vi "oa_Segment XY Graph Sub.vi"(7 "Reset? (F)":bool, 8 "error in (no error)":errorcluster, 9 "Limit range":bool, 10 "Segment settings":T1={"X start"=0.0, "X interval"=50.0, "X end"=6000.0} {"X end" min=0.0 format="%.2f"; "X interval" format="%.2f"; "X start" min=0.0 format="%.2f"}, 11 "XY Graph":cluster{"time/rev/rpm":dbl[], "magnitude":dbl[]}) -> (0 "error out":errorcluster, 3 "XY Graph out":cluster{"time/rev/rpm":dbl[], "magnitude":dbl[]})   [LabVIEW 2017, in "SoundVib_Resampling.lvlib"]
uses:
  <vilib>/addons/Sound and Vibration/Order Analysis/Resample Order Tracking/SoundVib_Resampling.lvlib
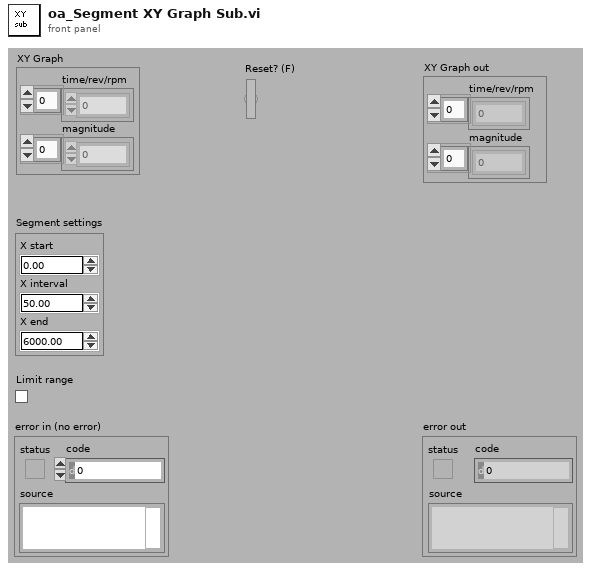
[diagram p1: front panel]
types:
  T1 = cluster{"X start":dbl, "X interval":dbl, "X end":dbl}
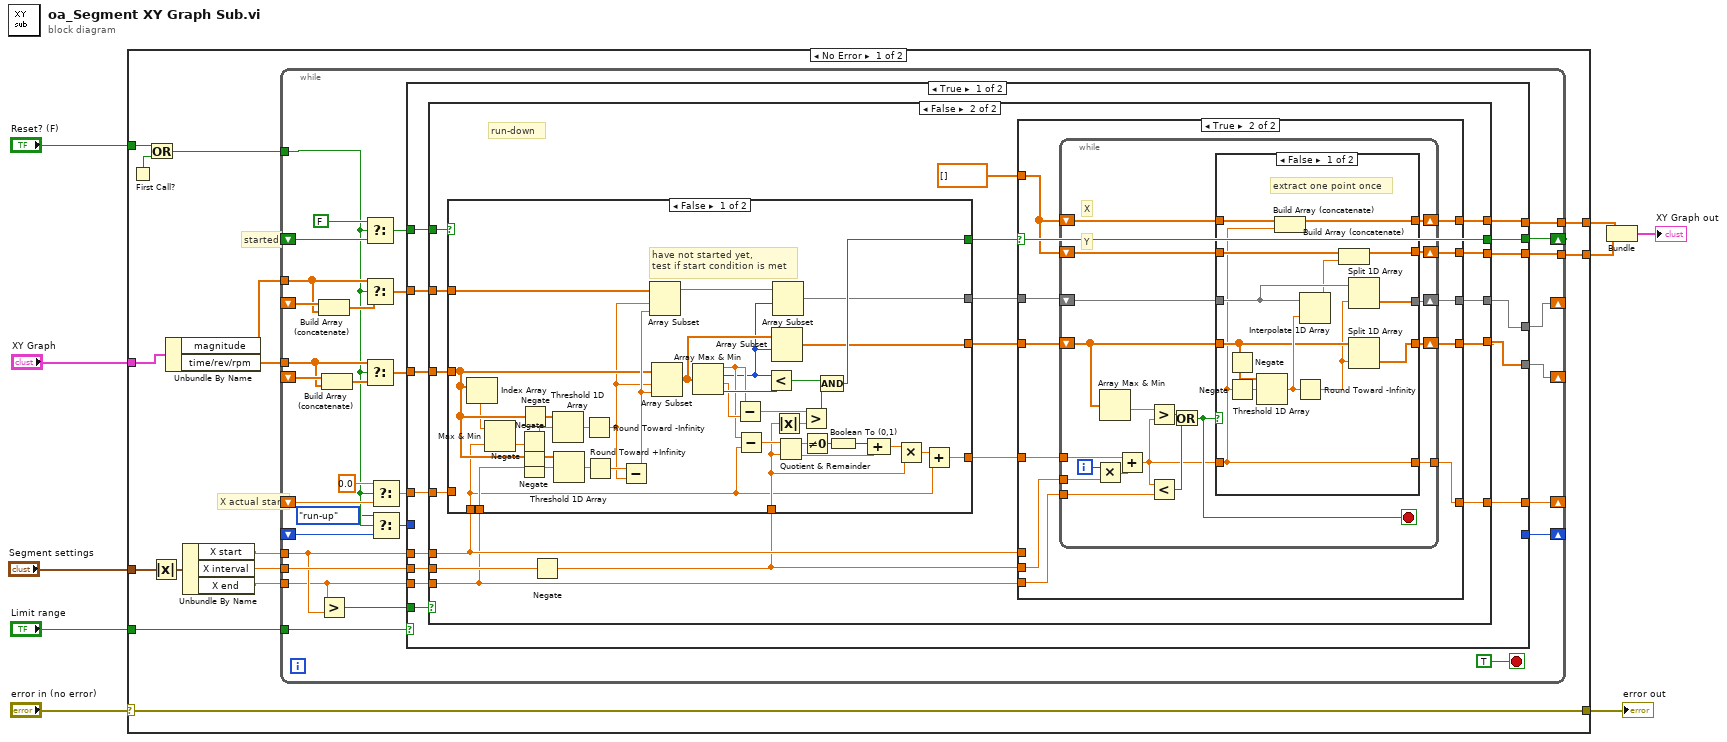
[diagram p0: block diagram]
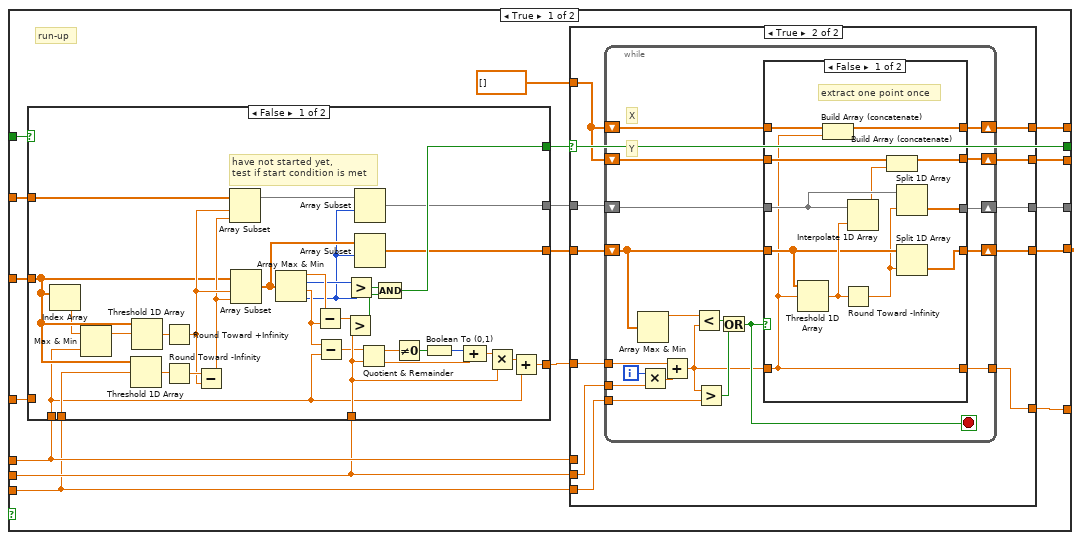
[diagram p2: hidden frame]
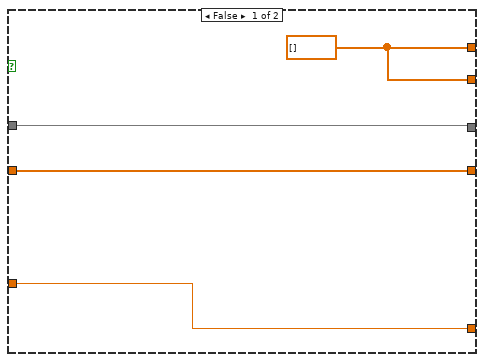
[diagram p3: hidden frame]
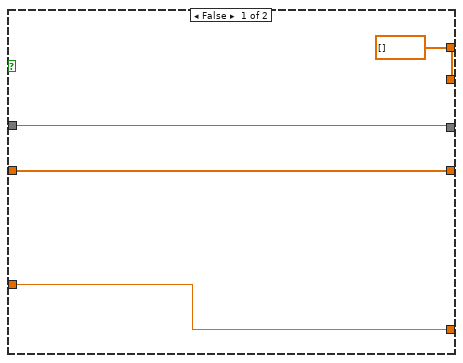
[diagram p6: hidden frame]
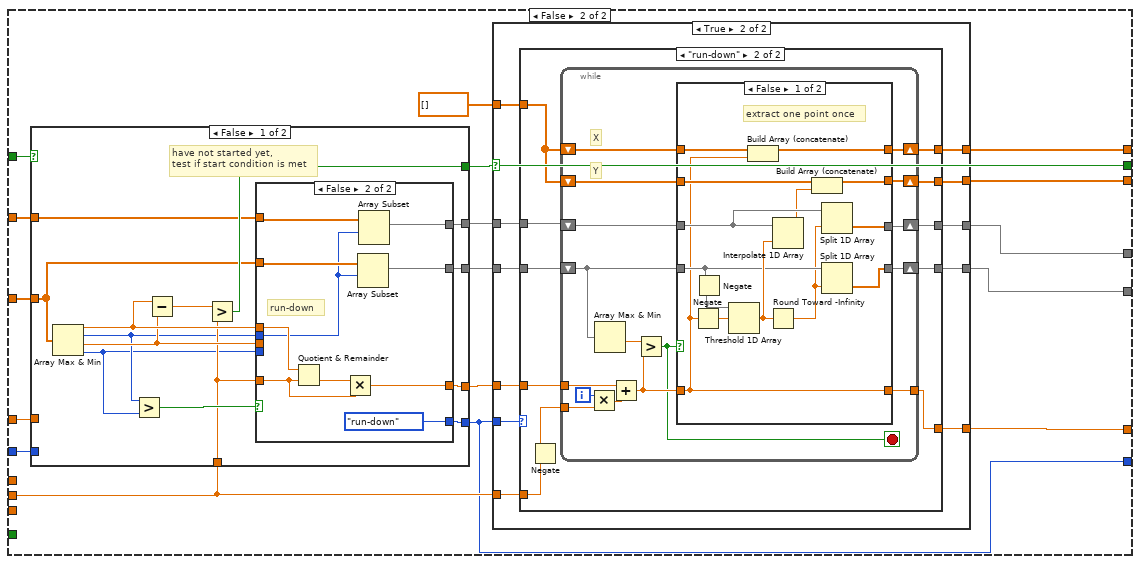
[diagram p9: hidden frame]
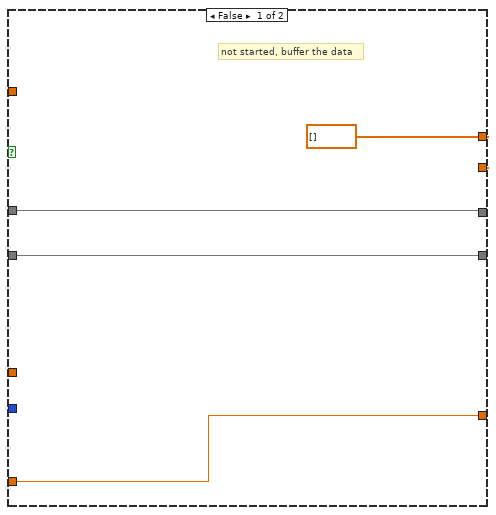
[diagram p10: hidden frame]
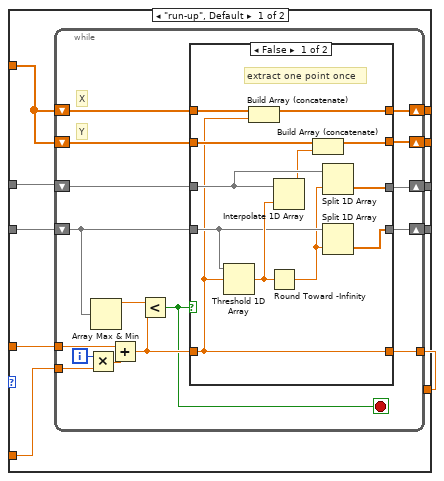
[diagram p11: hidden frame]
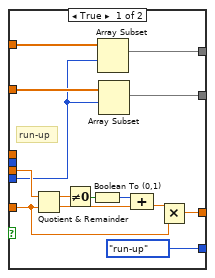
[diagram p14: hidden frame]
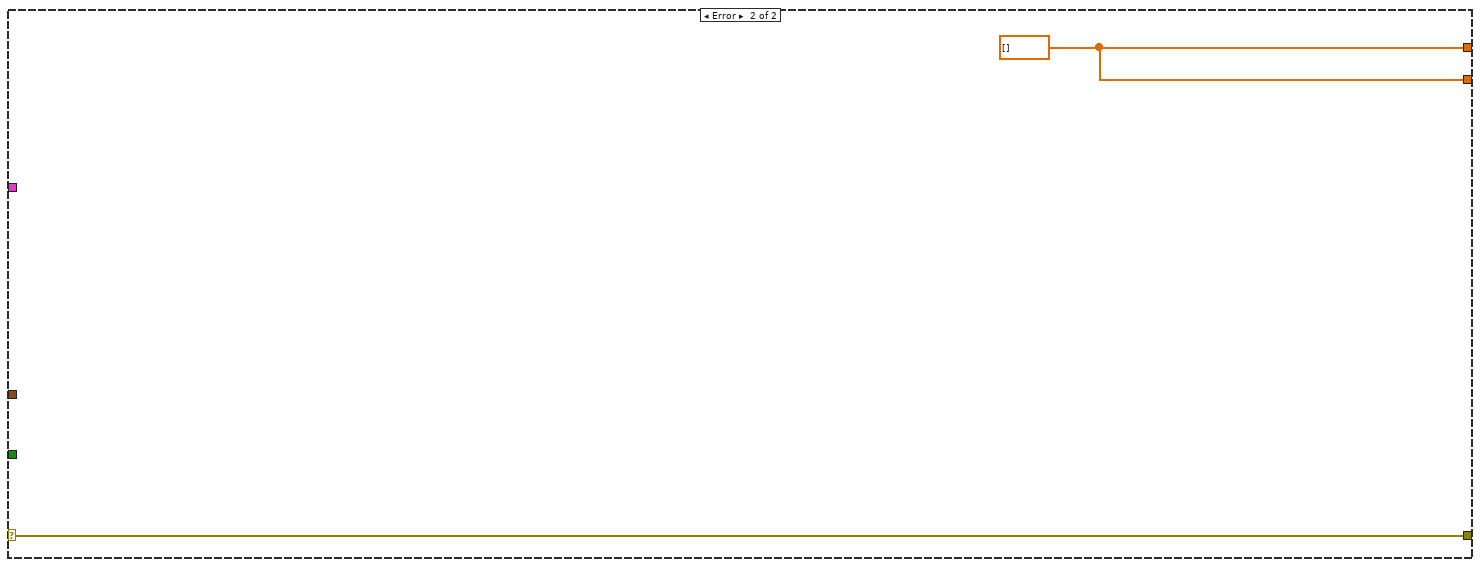
[diagram p16: hidden frame]
diagram:
  n1 = case shown="No Error" "error in (no error)" {
    selector: "error in (no error)" -> [w10 w451]
    tunnel: [w10 w451] -> w8
    tunnel: "Reset? (F)" -> [w24 _]
    tunnel: "Segment settings" -> [w17 _]
    tunnel: "Limit range" -> [w19 _]
    tunnel: "XY Graph" -> [w14 _]
    tunnel: [w12 w450] -> w3
    tunnel: [w11 w450] -> w2
    frame No Error {
      # "X actual start"
      # "started"
      n2 = First Call?() -> (First Call?: T/F=w23:bool)
      n3 = Or(x=w24, y=w23) -> (x .or. y?=w20:bool)
      n4 = Absolute Value(x=w17) -> (abs(x)=w16:T1)
      n5 = Unbundle By Name(w14) -> ("magnitude"=w13:dbl[], "time/rev/rpm"=w22:dbl[])
      n6 = Unbundle By Name(w16) -> ("X start"=w21:dbl, "X interval"=w18:dbl, "X end"=w15:dbl)
      n7 = while {
        tunnel: w22 -> [w52]
        tunnel: w21 -> [w37]
        shift-right: [w46] -> _
        shift-left: _ -> [w54]
        tunnel: w20 -> [w31]
        tunnel: w19 -> [w45]
        tunnel: w18 -> [w43]
        tunnel: w15 -> [w36]
        tunnel: w13 -> [w48]
        shift-right: [w47] -> _
        shift-left: _ -> [w50]
        shift-right: [w38] -> _
        shift-left: _ -> [w41]
        shift-right: [w33] -> _
        shift-left: _ -> [w34]
        shift-right: [w27] -> _
        shift-left: _ -> [w30]
        tunnel: [w26] -> w12
        tunnel: [w25] -> w11
        stop <- TRUE stop-if-true
        n8 = Build Array (concatenate)(w50, w48) -> (w49:dbl[])
        n9 = Greater?(x=w36, y=w37) -> (0:w44:bool)
        n10 = Build Array (concatenate)(w54, w52) -> (w53:dbl[])
        n11 = Select(t=FALSE, s=w31, f=w41) -> (s? t:f=w39:bool)
        n12 = Select(t=w48, s=w31, f=w49) -> (s? t:f=w42:dbl[])
        n13 = Select(t=w52, s=w31, f=w53) -> (s? t:f=w51:dbl[])
        n14 = Select(t=0.0, s=w31, f=w34) -> (s? t:f=w32:dbl)
        n15 = Select(t=enum16{"run-up", "run-down"}."run-up" ("process control"), s=w31, f=w30) -> (s? t:f=w28:enum16{"run-up", "run-down"})
        n16 = case shown="True" w45 {
          tunnel: w51 -> [w68 w300]
          tunnel: w42 -> [w62 w301]
          tunnel: [w57 w292] -> w47
          tunnel: [w56 w291] -> w46
          tunnel: w44 -> [w69 _]
          tunnel: w43 -> [w67 w294]
          tunnel: w39 -> [w66 w302]
          tunnel: [w65 w290] -> w38
          tunnel: w37 -> [w64 _]
          tunnel: w36 -> [w63 _]
          tunnel: w32 -> [w61 w299]
          tunnel: [w60 w289] -> w33
          tunnel: w28 -> [_ w298]
          tunnel: [_ w288] -> w27
          tunnel: [w59 w287] -> w26
          tunnel: [w58 w286] -> w25
          frame True {
            n17 = case shown="False" w69 {
              tunnel: w68 -> [w86 w191]
              tunnel: w67 -> [w78 w183]
              tunnel: w66 -> [w85 w190]
              tunnel: [w83 w188] -> w65
              tunnel: w64 -> [w79 w184]
              tunnel: w63 -> [w77 w182]
              tunnel: w62 -> [w84 w189]
              tunnel: w61 -> [w80 w185]
              tunnel: [w74 w179] -> w57
              tunnel: [w73 w178] -> w56
              tunnel: [w72 w177] -> w60
              tunnel: [w71 w175] -> w59
              tunnel: [w70 w174] -> w58
              frame True {
                # "run-up"
                n18 = case shown="False" w85 {
                  selector: w85 -> [_ w173]
                  tunnel: w86 -> [w141 w171]
                  tunnel: w78 -> [w151 _]
                  tunnel: [w164 w173] -> w83
                  tunnel: w79 -> [w139 _]
                  tunnel: w77 -> [w163 _]
                  tunnel: w84 -> [w159 w172]
                  tunnel: [w147 w170] -> w76
                  tunnel: [w145 w172] -> w82
                  tunnel: [w143 w171] -> w81
                  tunnel: w80 -> [_ w170]
                  frame False {
                    # "have not started yet,\ntest if start condition is met"
                    n19 = Index Array(array=w141) -> (element=w138:dbl)  [unwired: 1 in]
                    n20 = Max & Min(x=w138, y=w139) -> (max(x,y)=w140:dbl)  [unwired: 1 out]
                    n21 = Threshold 1D Array(2:w163, 3:w141) -> (0:w161:dbl)  [unwired: 1 in]
                    n22 = Threshold 1D Array(2:w140, 3:w141) -> (0:w162:dbl)  [unwired: 1 in]
                    n23 = Round Toward +Infinity(x=w162) -> (ceil(x): smallest int >= x=w158:dbl)
                    n24 = Round Toward -Infinity(1:w161) -> (0:w160:dbl)
                    n25 = Subtract(x=w160, y=w158) -> (x-y=w157:dbl)
                    n26 = Array Subset(array=w159, index=w158, length=w157) -> (w146:dbl[])
                    n27 = Array Subset(array=w141, index=w158, length=w157) -> (w144:dbl[])
                    n28 = Array Max & Min(array=w144) -> (max value=w169:dbl, max index (indices)=w167:i32, min value=w150:dbl, min index (indices)=w142:i32)
                    n29 = Subtract(x=w169, y=w150) -> (x-y=w168:dbl)
                    n30 = Subtract(x=w150, y=w139) -> (x-y=w149:dbl)
                    n31 = Greater?(x=w168, y=w151) -> (0:w165:bool)
                    n32 = Greater?(x=w167, y=w142) -> (0:w166:bool)
                    n33 = Array Subset(array=w146, index=w142) -> (w145:dbl[])  [unwired: 1 in]
                    n34 = Array Subset(array=w144, index=w142) -> (w143:dbl[])  [unwired: 1 in]
                    n35 = Quotient & Remainder(x=w149, y=w151) -> (x-y*floor(x/y)=w156:dbl, floor(x/y)=w153:dbl)
                    n36 = Compound Arithmetic op=AND(w166, w165) -> (w164:bool)
                    n37 = Not Equal To 0?(x=w156) -> (x != 0?=w155:bool)
                    n38 = Boolean To (0,1)(Boolean=w155) -> (0, 1=w154:i16)
                    n39 = Compound Arithmetic op=ADD(w154, w153) -> (w152:dbl)
                    n40 = Multiply(x=w152, y=w151) -> (x*y=w148:dbl)
                    n41 = Add(x=w148, y=w139) -> (x+y=w147:dbl)
                  }
                  frame True {
                    # "started"
                  }
                }
                n42 = case shown="True" w83 {
                  tunnel: w82 -> [w90 w101]
                  tunnel: w81 -> [w89 w100]
                  tunnel: w79 -> [_ _]
                  tunnel: w78 -> [_ w99]
                  tunnel: w77 -> [_ w98]
                  tunnel: w76 -> [w88 w97]
                  tunnel: dbl[] [] -> [_ w96]
                  tunnel: [w90 w95] -> w74
                  tunnel: [w89 w94] -> w73
                  tunnel: [w88 w93] -> w72
                  tunnel: [w87 w92] -> w71
                  tunnel: [w87 w91] -> w70
                  frame False {
                    w87 = dbl[] []
                  }
                  frame True {
                    n43 = while {
                      shift-right: [w117] -> w94
                      shift-left: w100 -> [w103]
                      tunnel: w99 -> [w120]
                      shift-right: [w118] -> w95
                      shift-left: w101 -> [w119]
                      shift-right: [w116] -> w92
                      shift-left: w96 -> [w115]
                      shift-right: [w114] -> w91
                      shift-left: w96 -> [w113]
                      tunnel: w98 -> [w112]
                      tunnel: w97 -> [w106]
                      tunnel: [w104] -> w93
                      i -> [w108]
                      stop <- w109 stop-if-true
                      # "Y"
                      # "X"
                      n44 = Array Max & Min(array=w103) -> (max value=w102:dbl)  [unwired: 3 out]
                      n45 = Multiply(x=w108, y=w120) -> (x*y=w107:dbl)
                      n46 = Add(x=w106, y=w107) -> (x+y=w105:dbl)
                      n47 = Less?(x=w102, y=w105) -> (x < y?=w111:bool)
                      n48 = Greater?(x=w105, y=w112) -> (0:w110:bool)
                      n49 = Or(x=w111, y=w110) -> (x .or. y?=w109:bool)
                      n50 = case shown="False" w109 {
                        tunnel: w103 -> [w131 w136]
                        tunnel: w105 -> [w121 w133]
                        tunnel: w119 -> [w130 w137]
                        tunnel: [w128 w137] -> w118
                        tunnel: [w127 w136] -> w117
                        tunnel: [w126 w134] -> w116
                        tunnel: w115 -> [w125 w134]
                        tunnel: [w123 w135] -> w114
                        tunnel: w113 -> [w122 w135]
                        tunnel: [w121 w133] -> w104
                        frame False {
                          # "extract one point once"
                          n51 = Threshold 1D Array(2:w121, 3:w131) -> (0:w132:dbl)  [unwired: 1 in]
                          n52 = Build Array (concatenate)(w125, w121) -> (w126:dbl[])
                          n53 = Round Toward -Infinity(1:w132) -> (0:w129:dbl)
                          n54 = Interpolate 1D Array(1:w132, 2:w130) -> (0:w124:dbl)
                          n55 = Build Array (concatenate)(w122, w124) -> (w123:dbl[])
                          n56 = Split 1D Array(array=w130, index=w129) -> (second subarray=w128:dbl[])  [unwired: 1 out]
                          n57 = Split 1D Array(array=w131, index=w129) -> (second subarray=w127:dbl[])  [unwired: 1 out]
                        }
                        frame True {
                          # "end of extract"
                        }
                      }
                    }
                  }
                }
              }
              frame False {
                # "run-down"
                n58 = Negate(x=w183) -> (-x=w176:dbl)
                n59 = case shown="False" w190 {
                  selector: w190 -> [_ w285]
                  tunnel: w191 -> [w253 w283]
                  tunnel: w176 -> [w255 _]
                  tunnel: [w277 w285] -> w188
                  tunnel: w184 -> [w252 _]
                  tunnel: w182 -> [w262 _]
                  tunnel: w189 -> [w274 w284]
                  tunnel: [w264 w282] -> w181
                  tunnel: [w257 w284] -> w187
                  tunnel: [w259 w283] -> w186
                  tunnel: w185 -> [_ w282]
                  frame False {
                    # "have not started yet,\ntest if start condition is met"
                    n60 = Index Array(array=w253) -> (element=w251:dbl)  [unwired: 1 in]
                    n61 = Max & Min(x=w251, y=w252) -> (min(x,y)=w248:dbl)  [unwired: 1 out]
                    n62 = Negate(x=w248) -> (-x=w247:dbl)
                    n63 = Negate(x=w253) -> (-x=w246:dbl[])
                    n64 = Negate(x=w262) -> (-x=w245:dbl)
                    n65 = Negate(x=w253) -> (-x=w249:dbl[])
                    n66 = Threshold 1D Array(2:w247, 3:w249) -> (0:w276:dbl)  [unwired: 1 in]
                    n67 = Threshold 1D Array(2:w245, 3:w246) -> (0:w275:dbl)  [unwired: 1 in]
                    n68 = Round Toward -Infinity(1:w276) -> (0:w250:dbl)
                    n69 = Round Toward +Infinity(x=w275) -> (ceil(x): smallest int >= x=w254:dbl)
                    n70 = Subtract(x=w254, y=w250) -> (x-y=w273:dbl)
                    n71 = Array Subset(array=w274, index=w250, length=w273) -> (w258:dbl[])
                    n72 = Array Subset(array=w253, index=w250, length=w273) -> (w260:dbl[])
                    n73 = Array Max & Min(array=w260) -> (max value=w263:dbl, max index (indices)=w256:i32, min value=w267:dbl, min index (indices)=w280:i32)
                    n74 = Subtract(x=w263, y=w267) -> (x-y=w281:dbl)
                    n75 = Subtract(x=w263, y=w252) -> (x-y=w266:dbl)
                    n76 = Less?(x=w256, y=w280) -> (x < y?=w279:bool)
                    n77 = Array Subset(array=w260, index=w256) -> (w259:dbl[])  [unwired: 1 in]
                    n78 = Array Subset(array=w258, index=w256) -> (w257:dbl[])  [unwired: 1 in]
                    n79 = Absolute Value(x=w255) -> (abs(x)=w261:dbl)
                    n80 = Quotient & Remainder(x=w266, y=w255) -> (x-y*floor(x/y)=w272:dbl, floor(x/y)=w269:dbl)
                    n81 = Greater?(x=w281, y=w261) -> (0:w278:bool)
                    n82 = Not Equal To 0?(x=w272) -> (x != 0?=w271:bool)
                    n83 = Compound Arithmetic op=AND(w279, w278) -> (w277:bool)
                    n84 = Boolean To (0,1)(Boolean=w271) -> (0, 1=w270:i16)
                    n85 = Compound Arithmetic op=ADD(w270, w269) -> (w268:dbl)
                    n86 = Multiply(x=w268, y=w255) -> (x*y=w265:dbl)
                    n87 = Add(x=w265, y=w252) -> (x+y=w264:dbl)
                  }
                  frame True {
                    # "started"
                  }
                }
                n88 = case shown="True" w188 {
                  tunnel: w187 -> [w195 w206]
                  tunnel: w186 -> [w194 w205]
                  tunnel: w184 -> [_ _]
                  tunnel: w176 -> [_ w204]
                  tunnel: w182 -> [_ w203]
                  tunnel: w181 -> [w193 w202]
                  tunnel: dbl[] [] -> [_ w201]
                  tunnel: [w195 w200] -> w179
                  tunnel: [w194 w199] -> w178
                  tunnel: [w193 w198] -> w177
                  tunnel: [w192 w197] -> w175
                  tunnel: [w192 w196] -> w174
                  frame False {
                    w192 = dbl[] []
                  }
                  frame True {
                    n89 = while {
                      shift-right: [w222] -> w199
                      shift-left: w205 -> [w208]
                      tunnel: w204 -> [w225]
                      shift-right: [w223] -> w200
                      shift-left: w206 -> [w224]
                      shift-right: [w221] -> w197
                      shift-left: w201 -> [w220]
                      shift-right: [w219] -> w196
                      shift-left: w201 -> [w218]
                      tunnel: w203 -> [w217]
                      tunnel: w202 -> [w211]
                      tunnel: [w209] -> w198
                      i -> [w213]
                      stop <- w214 stop-if-true
                      # "Y"
                      # "X"
                      n90 = Multiply(x=w213, y=w225) -> (x*y=w212:dbl)
                      n91 = Array Max & Min(array=w208) -> (min value=w207:dbl)  [unwired: 3 out]
                      n92 = Add(x=w211, y=w212) -> (x+y=w210:dbl)
                      n93 = Greater?(x=w207, y=w210) -> (0:w216:bool)
                      n94 = Less?(x=w210, y=w217) -> (x < y?=w215:bool)
                      n95 = Or(x=w216, y=w215) -> (x .or. y?=w214:bool)
                      n96 = case shown="False" w214 {
                        tunnel: w208 -> [w238 w243]
                        tunnel: w210 -> [w228 w240]
                        tunnel: w224 -> [w237 w244]
                        tunnel: [w235 w244] -> w223
                        tunnel: [w234 w243] -> w222
                        tunnel: [w233 w241] -> w221
                        tunnel: w220 -> [w232 w241]
                        tunnel: [w230 w242] -> w219
                        tunnel: w218 -> [w229 w242]
                        tunnel: [w228 w240] -> w209
                        frame False {
                          # "extract one point once"
                          n97 = Negate(x=w238) -> (-x=w227:dbl[])
                          n98 = Negate(x=w228) -> (-x=w226:dbl)
                          n99 = Threshold 1D Array(2:w226, 3:w227) -> (0:w239:dbl)  [unwired: 1 in]
                          n100 = Build Array (concatenate)(w232, w228) -> (w233:dbl[])
                          n101 = Round Toward -Infinity(1:w239) -> (0:w236:dbl)
                          n102 = Interpolate 1D Array(1:w239, 2:w237) -> (0:w231:dbl)
                          n103 = Build Array (concatenate)(w229, w231) -> (w230:dbl[])
                          n104 = Split 1D Array(array=w237, index=w236) -> (second subarray=w235:dbl[])  [unwired: 1 out]
                          n105 = Split 1D Array(array=w238, index=w236) -> (second subarray=w234:dbl[])  [unwired: 1 out]
                        }
                        frame True {
                          # "end of extract"
                        }
                      }
                    }
                  }
                }
              }
            }
          }
          frame False {
            n106 = case shown="False" w302 {
              selector: w302 -> [_ w449]
              tunnel: w300 -> [w410 w447]
              tunnel: w294 -> [w414 _]
              tunnel: [w418 w449] -> w290
              tunnel: w301 -> [w409 w448]
              tunnel: [w420 w446] -> w295
              tunnel: [w407 w448] -> w297
              tunnel: [w408 w447] -> w296
              tunnel: w299 -> [_ w446]
              tunnel: [w413 w445] -> w288
              tunnel: w298 -> [_ w445]
              frame False {
                # "have not started yet,\ntest if start condition is met"
                n107 = Array Max & Min(array=w410) -> (max value=w416:dbl, max index (indices)=w412:i32, min value=w415:dbl, min index (indices)=w411:i32)
                n108 = Greater?(x=w412, y=w411) -> (0:w417:bool)
                n109 = Subtract(x=w416, y=w415) -> (x-y=w419:dbl)
                n110 = Greater?(x=w419, y=w414) -> (0:w418:bool)
                n111 = case shown="False" w417 {
                  tunnel: [w434 w444] -> w420
                  tunnel: w416 -> [_ w442]
                  tunnel: w415 -> [w432 _]
                  tunnel: w414 -> [w433 w443]
                  tunnel: [enum16{"run-up", "run-down"}."run-up" ("process control") enum16{"run-up", "run-down"}."run-down" ("process control")] -> w413
                  tunnel: w412 -> [_ w435]
                  tunnel: w411 -> [w421 _]
                  tunnel: w410 -> [w425 w439]
                  tunnel: w409 -> [w423 w437]
                  tunnel: [w424 w438] -> w408
                  tunnel: [w422 w436] -> w407
                  frame True {
                    # "run-up"
                    n112 = Quotient & Remainder(x=w432, y=w433) -> (x-y*floor(x/y)=w431:dbl, floor(x/y)=w428:dbl)
                    n113 = Not Equal To 0?(x=w431) -> (x != 0?=w430:bool)
                    n114 = Boolean To (0,1)(Boolean=w430) -> (0, 1=w429:i16)
                    n115 = Array Subset(array=w423, index=w421) -> (w422:dbl[])  [unwired: 1 in]
                    n116 = Array Subset(array=w425, index=w421) -> (w424:dbl[])  [unwired: 1 in]
                    n117 = Compound Arithmetic op=ADD(w429, w428) -> (w427:dbl)
                    n118 = Multiply(x=w427, y=w433) -> (x*y=w434:dbl)
                  }
                  frame False {
                    # "run-down"
                    n119 = Quotient & Remainder(x=w442, y=w443) -> (floor(x/y)=w441:dbl)  [unwired: 1 out]
                    n120 = Multiply(x=w441, y=w443) -> (x*y=w444:dbl)
                    n121 = Array Subset(array=w439, index=w435) -> (w438:dbl[])  [unwired: 1 in]
                    n122 = Array Subset(array=w437, index=w435) -> (w436:dbl[])  [unwired: 1 in]
                  }
                }
              }
              frame True {
                # "started"
              }
            }
            n123 = case shown="True" w290 {
              tunnel: w288 -> [_ w317]
              tunnel: w297 -> [w306 w316]
              tunnel: w296 -> [w305 w315]
              tunnel: w295 -> [_ w314]
              tunnel: w294 -> [w304 w313]
              tunnel: dbl[] [] -> [_ w312]
              tunnel: [w306 w311] -> w292
              tunnel: [w305 w310] -> w291
              tunnel: [w304 w309] -> w289
              tunnel: [w303 w308] -> w287
              tunnel: [w303 w307] -> w286
              frame False {
                w303 = dbl[] []
                # "not started, buffer the data"
              }
              frame True {
                n124 = case shown="\"run-down\"" w317 {
                  tunnel: w316 -> [w327 w371]
                  tunnel: w315 -> [w326 w370]
                  tunnel: w313 -> [w325 w369]
                  tunnel: w314 -> [w324 w368]
                  tunnel: w312 -> [w323 w367]
                  tunnel: [w322 w366] -> w311
                  tunnel: [w321 w365] -> w310
                  tunnel: [w320 w361] -> w309
                  tunnel: [w319 w363] -> w308
                  tunnel: [w318 w362] -> w307
                  frame "run-up", Default {
                    n125 = while {
                      shift-right: [w340] -> w321
                      shift-left: w326 -> [w329]
                      tunnel: w325 -> [w343]
                      shift-right: [w341] -> w322
                      shift-left: w327 -> [w342]
                      shift-right: [w339] -> w319
                      shift-left: w323 -> [w338]
                      shift-right: [w337] -> w318
                      shift-left: w323 -> [w336]
                      tunnel: w324 -> [w333]
                      tunnel: [w331] -> w320
                      i -> [w335]
                      stop <- w330 stop-if-true
                      # "Y"
                      # "X"
                      n126 = Multiply(x=w335, y=w343) -> (x*y=w334:dbl)
                      n127 = Array Max & Min(array=w329) -> (max value=w328:dbl)  [unwired: 3 out]
                      n128 = Add(x=w333, y=w334) -> (x+y=w332:dbl)
                      n129 = Less?(x=w328, y=w332) -> (x < y?=w330:bool)
                      n130 = case shown="False" w330 {
                        tunnel: w329 -> [w354 w359]
                        tunnel: w332 -> [w344 w356]
                        tunnel: w342 -> [w353 w360]
                        tunnel: [w351 w360] -> w341
                        tunnel: [w350 w359] -> w340
                        tunnel: [w349 w357] -> w339
                        tunnel: w338 -> [w348 w357]
                        tunnel: [w346 w358] -> w337
                        tunnel: w336 -> [w345 w358]
                        tunnel: [w344 w356] -> w331
                        frame False {
                          # "extract one point once"
                          n131 = Threshold 1D Array(2:w344, 3:w354) -> (0:w355:dbl)  [unwired: 1 in]
                          n132 = Build Array (concatenate)(w348, w344) -> (w349:dbl[])
                          n133 = Round Toward -Infinity(1:w355) -> (0:w352:dbl)
                          n134 = Interpolate 1D Array(1:w355, 2:w353) -> (0:w347:dbl)
                          n135 = Build Array (concatenate)(w345, w347) -> (w346:dbl[])
                          n136 = Split 1D Array(array=w353, index=w352) -> (second subarray=w351:dbl[])  [unwired: 1 out]
                          n137 = Split 1D Array(array=w354, index=w352) -> (second subarray=w350:dbl[])  [unwired: 1 out]
                        }
                        frame True {
                          # "end of extract"
                        }
                      }
                    }
                  }
                  frame "run-down" {
                    n138 = Negate(x=w369) -> (-x=w364:dbl)
                    n139 = while {
                      shift-right: [w384] -> w365
                      shift-left: w370 -> [w373]
                      tunnel: w364 -> [w387]
                      shift-right: [w385] -> w366
                      shift-left: w371 -> [w386]
                      shift-right: [w383] -> w363
                      shift-left: w367 -> [w382]
                      shift-right: [w381] -> w362
                      shift-left: w367 -> [w380]
                      tunnel: w368 -> [w377]
                      tunnel: [w375] -> w361
                      i -> [w379]
                      stop <- w374 stop-if-true
                      # "Y"
                      # "X"
                      n140 = Multiply(x=w379, y=w387) -> (x*y=w378:dbl)
                      n141 = Array Max & Min(array=w373) -> (min value=w372:dbl)  [unwired: 3 out]
                      n142 = Add(x=w377, y=w378) -> (x+y=w376:dbl)
                      n143 = Greater?(x=w372, y=w376) -> (0:w374:bool)
                      n144 = case shown="False" w374 {
                        tunnel: w373 -> [w400 w405]
                        tunnel: w376 -> [w390 w402]
                        tunnel: w386 -> [w399 w406]
                        tunnel: [w397 w406] -> w385
                        tunnel: [w396 w405] -> w384
                        tunnel: [w395 w403] -> w383
                        tunnel: w382 -> [w394 w403]
                        tunnel: [w392 w404] -> w381
                        tunnel: w380 -> [w391 w404]
                        tunnel: [w390 w402] -> w375
                        frame False {
                          # "extract one point once"
                          n145 = Negate(x=w390) -> (-x=w389:dbl)
                          n146 = Negate(x=w400) -> (-x=w388:dbl[])
                          n147 = Threshold 1D Array(2:w389, 3:w388) -> (0:w401:dbl)  [unwired: 1 in]
                          n148 = Build Array (concatenate)(w394, w390) -> (w395:dbl[])
                          n149 = Round Toward -Infinity(1:w401) -> (0:w398:dbl)
                          n150 = Interpolate 1D Array(1:w401, 2:w399) -> (0:w393:dbl)
                          n151 = Build Array (concatenate)(w391, w393) -> (w392:dbl[])
                          n152 = Split 1D Array(array=w399, index=w398) -> (second subarray=w397:dbl[])  [unwired: 1 out]
                          n153 = Split 1D Array(array=w400, index=w398) -> (second subarray=w396:dbl[])  [unwired: 1 out]
                        }
                        frame True {
                          # "end of extract"
                        }
                      }
                    }
                  }
                }
              }
            }
          }
        }
      }
    }
    frame Error {
      w450 = dbl[] []
    }
  }
  "error out" <- w8
  n154 = Bundle(w3, w2) -> (→"XY Graph out":cluster{dbl[], dbl[]})  [unwired: 1 in]
